vi "Newmark-StagePosition.vi"(0 "Table VRN IN":refnum<visa-resource-name>, 7 "Bool Refnum":refnum<vi>, 11 "Error IN":errorcluster) -> (2 "X Axis":dbl, 3 "Y Axis":dbl, 4 "Table VRN OUT":refnum<visa-resource-name>, 6 "Error?":bool, 10 "OverTravel?":bool, 13 "T Axis":dbl, 14 "Z Axis":dbl, 15 "Error OUT":errorcluster)   [LabVIEW 2011]
uses:
  Comm/SerialCommError.vi
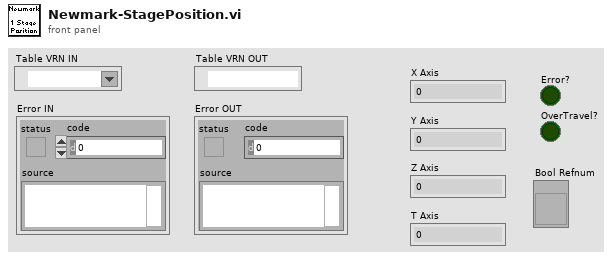
[diagram p1: front panel]
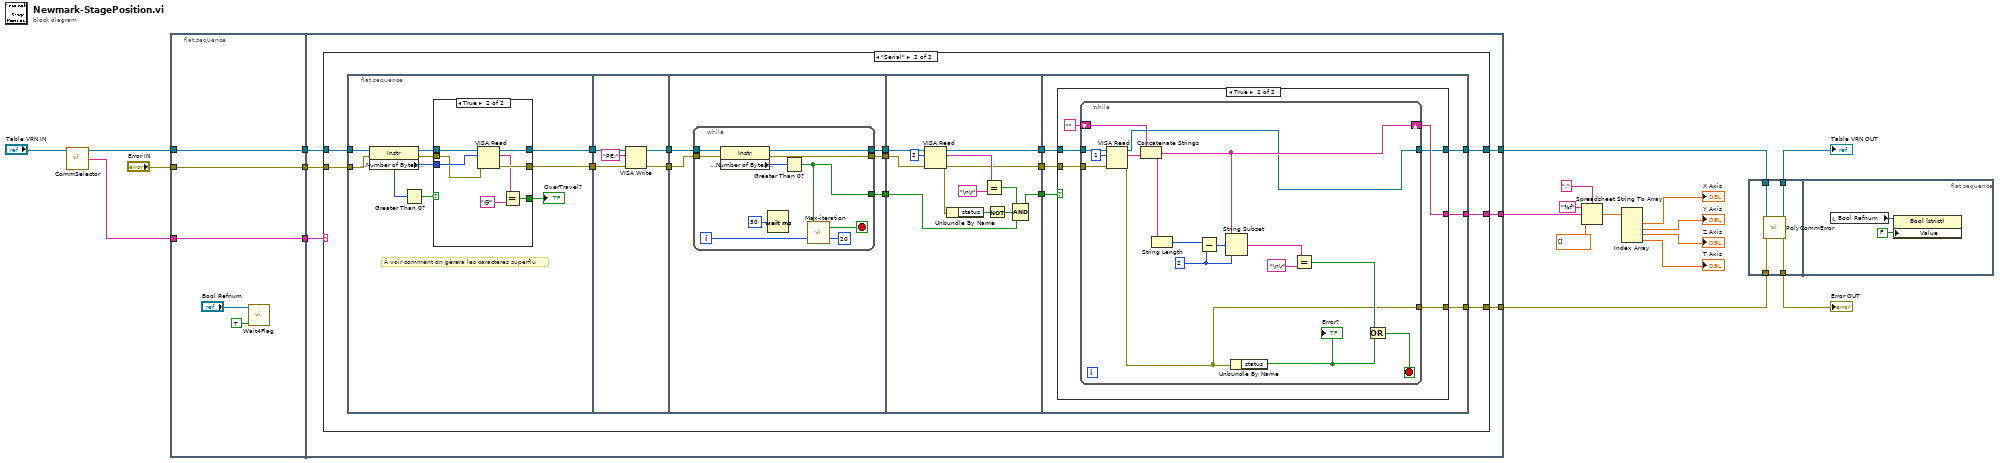
[diagram p0: block diagram]
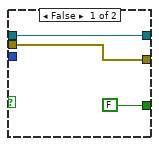
[diagram p3: hidden frame]
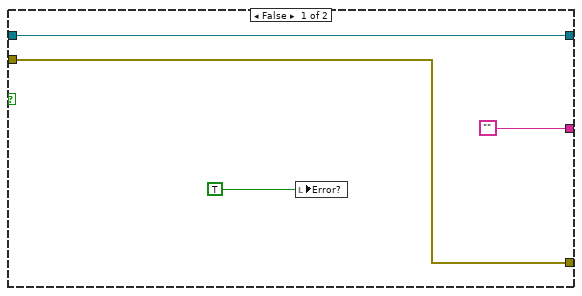
[diagram p4: hidden frame]
diagram:
  n1 = call "CommSelector.vi"("VISA resource name"="Table VRN IN") -> ("VISA resource name"=w11:refnum<visa-resource-name>, "CommType"=w9:string)  [unwired: 13 in]
  n2 = flat-sequence {
    tunnel: "Error IN" -> [w23]
    tunnel: w9 -> [w24]
    tunnel: w11 -> [w25]
    tunnel: [w25] -> w3
    tunnel: [w24] -> w2
    tunnel: [w23] -> w1
    tunnel: w3 -> [w30]
    tunnel: w2 -> [w29]
    tunnel: w1 -> [w28]
    tunnel: [w31] -> w20
    tunnel: [w27] -> w7
    tunnel: [w26] -> w6
    frame #0 {
      n3 = call "Wait4Flag.vi"("Raise Flag ?"=TRUE, "Ctl Refnum IN"="Bool Refnum") -> ()  [unwired: 8 in, 2 out]
    }
    frame #1 {
      n4 = case shown="\"Serial\"" w29 {
        tunnel: ["" w39] -> w31
        tunnel: [w34 w38] -> w26
        tunnel: [w33 w37] -> w27
        tunnel: w28 -> [w34 w36]
        tunnel: w30 -> [w33 w35]
        frame "Unknown", Default {
        }
        frame "Serial" {
          n5 = flat-sequence {
            tunnel: [w58] -> w49
            tunnel: [w57] -> w48
            tunnel: w35 -> [w56]
            tunnel: w36 -> [w55]
            tunnel: [w73] -> w47
            tunnel: [w72] -> w46
            tunnel: w49 -> [w71]
            tunnel: w48 -> [w70]
            tunnel: w47 -> [w79]
            tunnel: w46 -> [w78]
            tunnel: [w77] -> w45
            tunnel: [w76] -> w44
            tunnel: [w75] -> w43
            tunnel: w45 -> [w100]
            tunnel: w44 -> [w99]
            tunnel: [w95] -> w42
            tunnel: w43 -> [w93]
            tunnel: [w98] -> w41
            tunnel: [w91] -> w40
            tunnel: w42 -> [w106]
            tunnel: w41 -> [w107]
            tunnel: w40 -> [w104]
            tunnel: [w105] -> w39
            tunnel: [w103] -> w38
            tunnel: [w102] -> w37
            frame #0 {
              # "À voir comment on gèrera les caractères superflu"
              n6 = property class="Instr"(reference=w56, error in=w55) -> (reference out=w51:refnum<visa-resource-name>, error out=w52:errorcluster, "Serial Settings:Number of Bytes at Serial Port"=w53:u32)
              n7 = Greater Than 0?(x=w53) -> (x > 0?=w54:bool)
              n8 = case shown="True" w54 {
                tunnel: [w61 w69] -> w58
                tunnel: [w60 w68] -> w57
                tunnel: w53 -> [_ w67]
                tunnel: w52 -> [w60 w66]
                tunnel: w51 -> [w61 w65]
                tunnel: [FALSE w62] -> w50
                frame False {
                }
                frame True {
                  n9 = VISA Read(VISA resource name=w65, byte count=w67, error in (no error)=w66) -> (VISA resource name out=w69:refnum<visa-resource-name>, read buffer=w64:string, error out=w68:errorcluster)  [unwired: 1 out]
                  n10 = Equal?(x=w64, y="@") -> (x = y?=w62:bool)
                }
              }
              "OverTravel?" <- w50
            }
            frame #1 {
              n11 = VISA Write(VISA resource name=w71, write buffer="PE;", error in (no error)=w70) -> (VISA resource name out=w73:refnum<visa-resource-name>, error out=w72:errorcluster)  [unwired: 1 out]
            }
            frame #2 {
              n12 = while {
                tunnel: w79 -> [w85]
                tunnel: w78 -> [w84]
                tunnel: [w82] -> w75
                tunnel: [w81] -> w77
                tunnel: [w80] -> w76
                i -> [w88]
                stop <- w89 stop-if-true
                n13 = property class="Instr"(reference=w85, error in=w84) -> (reference out=w81:refnum<visa-resource-name>, error out=w80:errorcluster, "Serial Settings:Number of Bytes at Serial Port"=w83:u32)
                n14 = Wait (ms)(milliseconds to wait=u32 50) -> ()  [unwired: 1 out]
                n15 = Greater Than 0?(x=w83) -> (x > 0?=w82:bool)
                n16 = call "Max-iteration.vi"("i max"=20, "i act"=w88, "Valeur entrante"=w82) -> ("break ?"=w89:bool)
              }
            }
            frame #3 {
              n17 = VISA Read(VISA resource name=w100, byte count=u32 2, error in (no error)=w99) -> (VISA resource name out=w98:refnum<visa-resource-name>, read buffer=w96:string, error out=w95:errorcluster)  [unwired: 1 out]
              n18 = Unbundle By Name(w95) -> ("status"=w92:bool)
              n19 = Equal?(x=w96, y="\n\r") -> (x = y?=w94:bool)
              n20 = Not(x=w92) -> (.not. x?=w90:bool)
              n21 = Compound Arithmetic op=AND(w94, w90, w93) -> (w91:bool)
            }
            frame #4 {
              n22 = case shown="True" w104 {
                tunnel: w107 -> [w109 w117]
                tunnel: w106 -> [w110 w116]
                tunnel: ["" w114] -> w105
                tunnel: [w110 w113] -> w103
                tunnel: [w109 w112] -> w102
                frame False {
                  n23 = local write "Error?"(TRUE ("Error?")) -> ()
                }
                frame True {
                  n24 = while {
                    tunnel: w117 -> [w133]
                    tunnel: w116 -> [w132]
                    shift-right: [w126] -> w114
                    shift-left: "" -> [w125]
                    tunnel: [w119] -> w113
                    tunnel: [w118] -> w112
                    stop <- w120 stop-if-true
                    w129 = 2 ("y")
                    n25 = VISA Read(VISA resource name=w133, byte count=u32 1, error in (no error)=w132) -> (VISA resource name out=w118:refnum<visa-resource-name>, read buffer=w124:string, error out=w119:errorcluster)  [unwired: 1 out]
                    n26 = Concatenate Strings(w125, w124) -> (w126:string)
                    n27 = String Length(string=w126) -> (length=w123:i32)
                    n28 = Subtract(x=w123, y=w129) -> (x-y=w130:i32)
                    n29 = String Subset(string=w126, offset (0)=w130, length (rest)=w129) -> (substring=w128:string)
                    n30 = Unbundle By Name(w119) -> ("status"=w122:bool)
                    "Error?" <- w122
                    n31 = Equal?(x=w128, y="\n\r") -> (x = y?=w121:bool)
                    n32 = Or(x=w121, y=w122) -> (x .or. y?=w120:bool)
                  }
                }
              }
            }
          }
        }
      }
    }
  }
  n33 = Spreadsheet String To Array(delimiter (Tab)=",", format string="%f", spreadsheet string=w20, array type (2D Dbl)=dbl[] []) -> (array=w16:dbl[])
  n34 = Index Array(array=w16) -> (element #1=→"X Axis":dbl, element #2=→"Y Axis":dbl, element #3=→"Z Axis":dbl, element #4=→"T Axis":dbl)  [unwired: 4 in]
  n35 = flat-sequence {
    tunnel: w7 -> [w136]
    tunnel: w6 -> [w137]
    tunnel: [w135] -> w4
    tunnel: [w134] -> w5
    frame #0 {
      n36 = call-poly "PolyCommError.vi"("VISA IN"=w136, "error IN"=w137) -> ("VISA OUT"=w135:refnum<visa-resource-name>, "error OUT"=w134:errorcluster)  [unwired: 11 in, 1 out]
    }
    frame #1 {
      n37 = local read "Bool Refnum"() -> (w139:refnum<vi>)
      n38 = property class="Bool (strict)"(reference=w139, "Value"=FALSE) -> ()  [unwired: 1 in, 2 out]
    }
  }
  "Table VRN OUT" <- w4
  "Error OUT" <- w5
